vi "Sort & Remove Duplicate Edges.vi"(9 "Rotations":u16, 10 "Pattern":T1) -> (2 "Pattern":T1)   [LabVIEW 2017, in "Engine Simulation Toolkit System Explorer.lvlib"]
uses:
  Engine Simulation Toolkit System Explorer.lvlib
  Digital Pattern Expanded.ctl
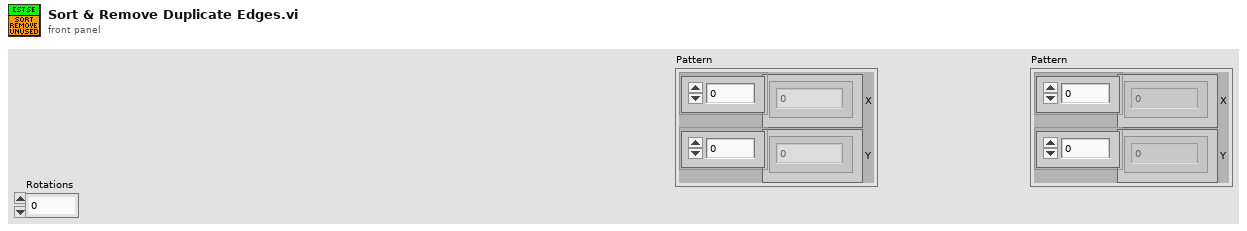
[diagram p1: front panel]
types:
  T1 = typedef "Engine Simulation Toolkit System Explorer.lvlib/Digital Pattern Expanded.ctl" = cluster{"X":dbl[], "Y":dbl[]}
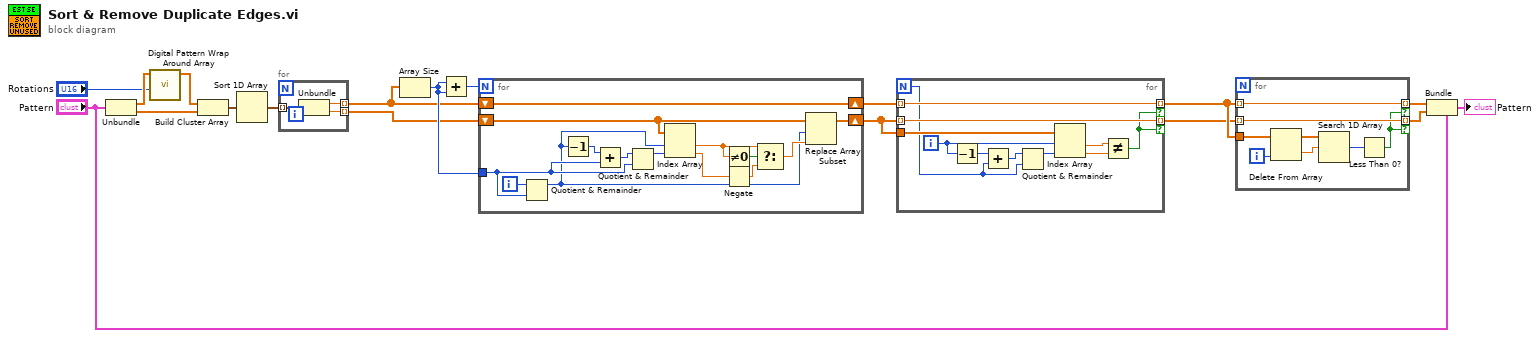
[diagram p0: block diagram]
diagram:
  n1 = Unbundle("Pattern") -> ("X"=w14:dbl[], "Y"=w16:dbl[])
  n2 = call "Digital Pattern Wrap Around Array.vi"("Rotations"="Rotations", "x"=w14) -> ("x"=w13:dbl[])  [unwired: 9 in]
  n3 = Build Cluster Array(w13, w16) -> (w15:cluster{dbl, "Numeric Control":dbl}[])
  n4 = Sort 1D Array(array=w15) -> (sorted array=w9:cluster{dbl, "Numeric Control":dbl}[])
  n5 = for {
    tunnel: w9 -> [w21] mode=indexing
    tunnel: [w20] -> w4 mode=indexing
    tunnel: [w19] -> w3 mode=indexing
    n6 = Unbundle(w21) -> (w20:dbl, "Numeric Control"=w19:dbl)
  }
  n7 = Array Size(array=w4) -> (size(s)=w7:i32)
  n8 = Add(x=w7, y=w7) -> (x+y=w8:i32)
  n9 = for {
    N: w8 -> [_]
    shift-right: [w25] -> w6
    shift-left: w4 -> [w25]
    shift-right: [w32] -> w5
    shift-left: w3 -> [w31]
    tunnel: w7 -> [w23]
    i -> [w33]
    n10 = Quotient & Remainder(x=w33, y=w23) -> (x-y*floor(x/y)=w22:i32)  [unwired: 1 out]
    n11 = Decrement(x=w22) -> (x-1=w30:i32)
    n12 = Add(x=w30, y=w23) -> (x+y=w24:i32)
    n13 = Quotient & Remainder(x=w24, y=w23) -> (x-y*floor(x/y)=w29:i32)  [unwired: 1 out]
    n14 = Index Array(array=w31, index #1=w22, index #2=w29) -> (element #1=w28:dbl, element #2=w27:dbl)
    n15 = Not Equal To 0?(x=w28) -> (x != 0?=w35:bool)
    n16 = Negate(x=w27) -> (-x=w34:dbl)
    n17 = Select(t=w28, s=w35, f=w34) -> (s? t:f=w26:dbl)
    n18 = Replace Array Subset(array=w31, new element=w26, index=w22) -> (w32:dbl[])
  }
  n19 = for {
    N -> [w36]
    tunnel: w6 -> [w45] mode=indexing
    tunnel: [w45] -> w2 mode=indexing if=w39
    tunnel: w5 -> [w44] mode=indexing
    tunnel: [w44] -> w1 mode=indexing if=w39
    tunnel: w5 -> [w42]
    i -> [w43]
    n20 = Decrement(x=w43) -> (x-1=w38:i32)
    n21 = Add(x=w38, y=w36) -> (x+y=w37:i32)
    n22 = Quotient & Remainder(x=w37, y=w36) -> (x-y*floor(x/y)=w46:i32)  [unwired: 1 out]
    n23 = Index Array(array=w42, index #1=w43, index #2=w46) -> (element #1=w41:dbl, element #2=w40:dbl)
    n24 = Not Equal?(x=w41, y=w40) -> (x != y?=w39:bool)
  }
  n25 = for {
    tunnel: w2 -> [w54]
    tunnel: [w49] -> w11 mode=indexing if=w47
    tunnel: w2 -> [w49] mode=indexing
    tunnel: w1 -> [w48] mode=indexing
    tunnel: [w48] -> w10 mode=indexing if=w47
    i -> [w53]
    n26 = Delete From Array(array=w54, index=w53) -> (deleted portion=w50:dbl, array with subset deleted=w52:dbl[])  [unwired: 1 in]
    n27 = Search 1D Array(1D array=w52, element=w50) -> (index of element=w51:i32)  [unwired: 1 in]
    n28 = Less Than 0?(x=w51) -> (x < 0?=w47:bool)
  }
  n29 = Bundle(cluster="Pattern", "X"=w11, "Y"=w10) -> (→"Pattern":T1)
